vi "GetRefNumTypes.vi"(8 "error in (no error)":errorcluster, 11 "Control in":refnum<vi>) -> (0 "error out":errorcluster, 2 "RefNumType":string, 3 "Control Ref Out":refnum<vi>)   [LabVIEW 2014]
doc: "This subVI retrieves the refnum type from a lookup table"
panel:
  in  "Refnum Types":string[][](array[string])=[["3412", "App Refnum"], ["3422", "VIRefNum"], ["3419", "Ctl Refnum"], ["3406", "Occurrence Refnum"], ["3413", "Menu Refnum"], ["3407", "TCP Network Connection Refnum"], ["3418", "UDP Network Connection Refnum"], ["3450", "IrDA Refnum"], ["3468", "Bluetooth Refnum"], ["3417", "DataSocket Refnum"], ["3408", "Byte Stream File Refnum"], ["3402", "Data Log File Refnum"], ["3410", "Automation Refnum"], ["3441", ".NET Refnum"], ["3435", "Event Callback"]]
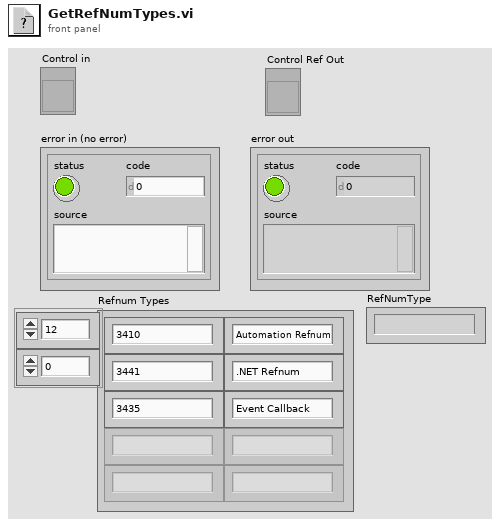
[diagram p1: front panel]
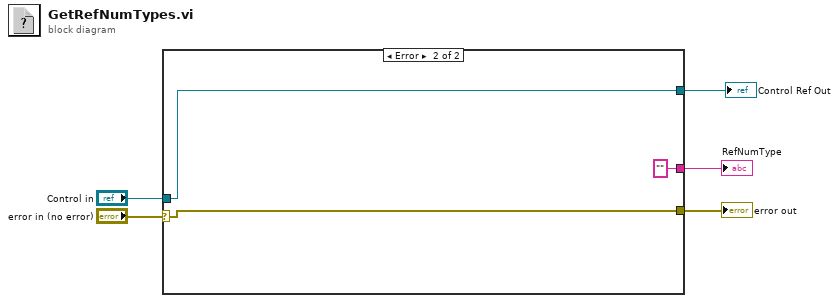
[diagram p0: block diagram]
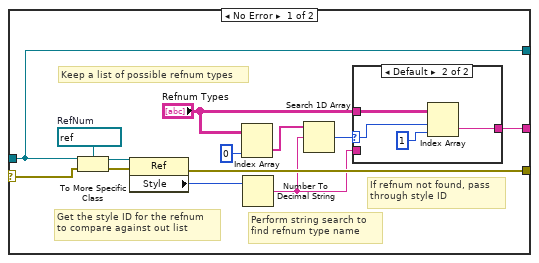
[diagram p2: hidden frame]
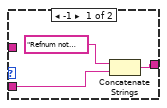
[diagram p3: hidden frame]
diagram:
  n1 = case shown="Error" "error in (no error)" {
    selector: "error in (no error)" -> [w14 w28]
    tunnel: [w16 w28] -> w5
    tunnel: "Control in" -> [w6 w26]
    tunnel: [w9 "" ("String")] -> w2
    tunnel: [w6 w26] -> w1
    frame No Error {
      w18 = refnum<vi> refnum  # RefNum
      # "If refnum not found, pass\nthrough style ID"
      # "Perform string search to \nfind refnum type name"
      # "Get the style ID for the refnum \nto compare against out list"
      # "Keep a list of possible refnum types"
      n2 = To More Specific Class(target class=w18, reference=w6, error in=w14) -> (specific class reference=w17:refnum<vi>, error out=w15:errorcluster)
      n3 = property class="Ref"(reference=w17, error in=w15) -> (error out=w16:errorcluster, "Style"=w11:u32)  [unwired: 1 out]
      n4 = Index Array(array="Refnum Types", index (col)=0 ("disabled index (col)")) -> (element=w12:string[])  [unwired: 1 in]
      n5 = Number To Decimal String(number=w11) -> (decimal integer string=w7:string)  [unwired: 1 in]
      n6 = Search 1D Array(1D array=w12, element=w7) -> (index of element=w8:i32)  [unwired: 1 in]
      n7 = case shown="Default" w8 {
        selector: w8 -> [_ w22]
        tunnel: "Refnum Types" -> [_ w24]
        tunnel: [w20 w23] -> w9
        tunnel: w7 -> [w19 _]
        frame -1 {
          n8 = Concatenate Strings("Refnum not found: " ("String"), w19) -> (w20:string)
        }
        frame Default {
          n9 = Index Array(array=w24, index (row)=w22, index (col)=1) -> (element=w23:string)
        }
      }
    }
    frame Error {
    }
  }
  "error out" <- w5
  "RefNumType" <- w2
  "Control Ref Out" <- w1
